vi "Чтение из тдма.vi"(10 "tdm":string, 11 "Канал":string) -> (3 "data":dbl[](array[numeric]))   [LabVIEW 2011]
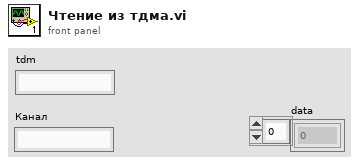
[diagram p1: front panel]
types:
  T1 = enum16{"big-endian, network order", "native, host order", "little-endian"}
  T2 = enum16{"open", "open or create", "create or replace", "create", "open (read-only)"}
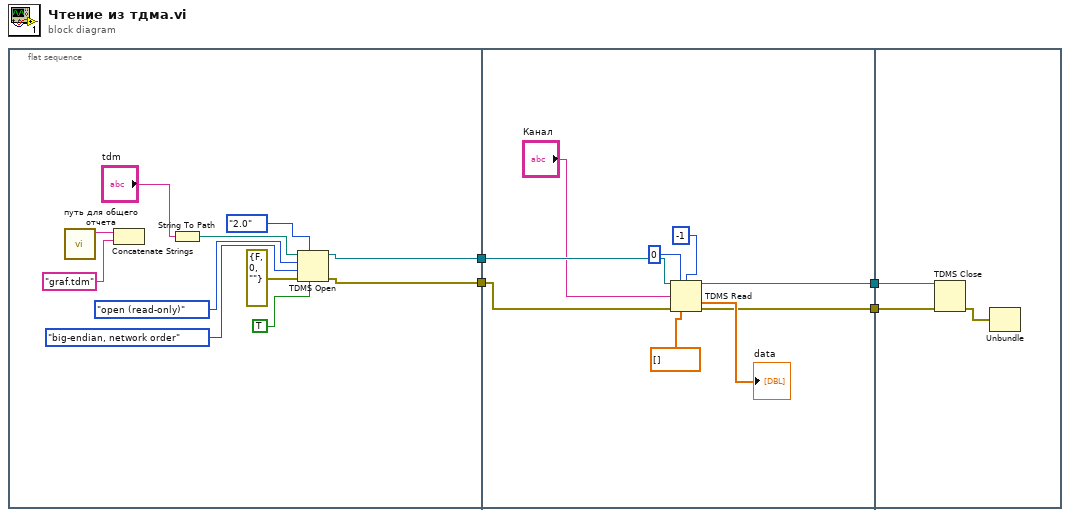
[diagram p0: block diagram]
diagram:
  n1 = flat-sequence {
    tunnel: [w7] -> w4
    tunnel: [w6] -> w3
    tunnel: w4 -> [w23]
    tunnel: w3 -> [w22]
    tunnel: [w18] -> w2
    tunnel: [w17] -> w1
    tunnel: w2 -> [w27]
    tunnel: w1 -> [w26]
    frame #0 {
      n2 = call "путь для общего отчета.vi"() -> ("path_out 2"=w15:string)  [unwired: 11 in]
      n3 = Concatenate Strings(w15, "graf.tdm") -> ()  [unwired: 1 out]
      n4 = String To Path(string="tdm") -> (path=w8:path)
      n5 = TDMS Open(6:TRUE ("disable buffering? (T)"), 7:enum16{"1.0", "2.0"}."2.0" ("file format version (2.0)"), 8:errorcluster {"status"=FALSE, "code"=0, "source"=""} ("error in (no error)"), 9:T1."big-endian, network order" ("byte order (2:little-endian)"), 10:T2."open (read-only)" ("operation (0:open)"), 11:w8) -> (0:w6:errorcluster, 3:w7:refnum<k34>)
    }
    frame #1 {
      n6 = TDMS Read(0:w23, 1:i64 0 ("offset (0)"), 2:i64 -1 ("count (-1: all)"), 7:"Канал", 11:w22, 12:dbl[] []) -> (4:w18:refnum<k34>, 10:→"data":dbl[], 15:w17:errorcluster)  [unwired: 2 in, 3 out]
    }
    frame #2 {
      n7 = TDMS Close(8:w26, 11:w27) -> (0:w25:errorcluster)  [unwired: 1 out]
      n8 = Unbundle(w25) -> ()  [unwired: 3 out]
    }
  }
